vi "AsyncEngine.CANProtectionAndCounter.vi"(10 "Parameters":variant, 11 "Process":refnum<class "Process.lvclass">) -> ()   [LabVIEW 2015, in "Protection and Rolling Counter Addon Engine.lvlib"]
uses:
  Protection and Rolling Counter Addon Engine.lvlib
  <vilib>/NI/NIVS Inline Async API/_VS Inline Async API/Process/Process.lvclass
  Types/RT Async Engine Variables.ctl
  Types/RT Frame Settings.ctl
  Shared/Types/Exported Frame Type.ctl
  Types/RT Protection Configuration.ctl
  Shared/Types/Protection Type.ctl
  Shared/Types/InputChannelConfiguration.ctl
  Types/RT Counter Settings.ctl
  Shared/Types/Event Trigger Type.ctl
  Types/RT Data References.ctl
  <vilib>/NI/NIVS Inline Async API/_Data Access Engine/Data Access Engine/Types/Write.DVR.ctl
  <vilib>/NI/NIVS Inline Async API/_Data Access Engine/Access Type Classes/Write/Write.lvclass
  <vilib>/NI/NIVS Inline Async API/_Data Access Engine/Data Access Engine/Types/Read.DVR.ctl
  <vilib>/NI/NIVS Inline Async API/_Data Access Engine/Access Type Classes/Read/Read.lvclass
  <vilib>/NI/NIVS Inline Async API/_VS Inline Async API/Process/Process.lvclass/Process.ctl
  <vilib>/Platform/TimedLoop/XDataNode/timing_clust.ctl
  <vilib>/Platform/TimedLoop/XDataNode/nitl_modes.ctl
  <vilib>/Platform/TimedLoop/XDataNode/wakeup.ctl
  <vilib>/NI/NIVS Inline Async API/_Data Access Engine/Access Type Classes/Read/Read.lvclass/Read.ctl
  <vilib>/NI/NIVS Inline Async API/_Data Access Engine/Access Type Classes/Write/Write.lvclass/Write.ctl
  <vilib>/NI/NIVS Inline Async API/_VS Inline Async API/Process/Data Member Access/Read Data Access.vi
  <vilib>/NI/NIVS Inline Async API/_VS Inline Async API/Error Handling Process/SubVIs/Error.ConvertArray.vi
  <vilib>/NI/NIVS Inline Async API/_Data Access Engine/Data Access Engine/Methods/Data.Processes.Execute.vi
  <vilib>/NI/NIVS Inline Async API/_Data Access Engine/Data Access Engine/Methods/Write.Data.Buffer.vi
  SubVIs/Determine Transmission.vi
  SubVIs/Determine Periodic.vi
  <vilib>/NI/NIVS Inline Async API/_Data Access Engine/Data Access Engine/Methods/Write.Data.Commit.vi
  <vilib>/NI/NIVS Inline Async API/_Data Access Engine/Data Access Engine/Methods/Write.Data.vi
  <vilib>/NI/NIVS Inline Async API/_Data Access Engine/Data Access Engine/Methods/Read.Data.Detect.vi
  <vilib>/NI/NIVS Inline Async API/_Data Access Engine/Access Type Classes/Write/Write.Buffer.vi
  <vilib>/NI/NIVS Inline Async API/_Data Access Engine/Access Type Classes/Write/Write.Commit.vi
  <vilib>/NI/NIVS Inline Async API/_Data Access Engine/Access Type Classes/Write/Write.ProcessData.vi
  <vilib>/NI/NIVS Inline Async API/_Data Access Engine/Access Type Classes/Read/Read.ProcessData.Detect.vi
  <vilib>/xnet/xnet.llb/XNET Write.vi
  <vilib>/xnet/xnet.llb/XNET Write (Frame CAN).vi
  <vilib>/xnet/xnet.llb/XNET Convert.vi
  <vilib>/xnet/xnet.llb/XNET Convert (Signal to Frame CAN).vi
  <vilib>/xnet/xnet.llb/XNET Convert (Signal to Frame Raw).vi
  <vilib>/NI/NIVS Inline Async API/_Data Access Engine/Data Access Engine/Methods/Write.Lookup.vi
  <vilib>/NI/NIVS Inline Async API/_Data Access Engine/Data Access Engine/Methods/Read.Lookup.vi
  Shared/SubVIs/GUID Lookup.vi
  <vilib>/platform/TimedLoop/XDataNode/XDataNode.xnode
  <vilib>/NI/NIVS Inline Async API/_Data Access Engine/Data Access Engine/Data Access Engine.lvclass
  Shared/Protection and Rolling Counter Addon Shared.lvlib
  <vilib>/NI VeriStand/Custom Device Tools/Custom Device Utility Library/Custom Device Utility Library.lvlib
  <vilib>/Platform/TimedLoop/XDataNode/XDNodeRunTimeDep.lvlib
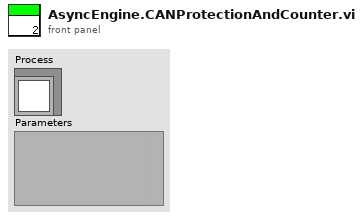
[diagram p1: front panel]
types:
  T1 = typedef "Protection and Rolling Counter Addon Engine.lvlib/RT Data References.ctl" = cluster{"ProtectionsAndCounters.Ref":T2, "Signals.Ref":T3, "Status.Ref":T2}
  T2 = typedef "Data Access Engine.lvlib/Data Access Engine.lvclass/Write.DVR.ctl" = refnum<data-value>
  T3 = typedef "Data Access Engine.lvlib/Data Access Engine.lvclass/Read.DVR.ctl" = refnum<data-value>
  T4 = typedef "Protection and Rolling Counter Addon Engine.lvlib/RT Async Engine Variables.ctl" = cluster{"Priority":i32, "CAN Session":refnum<k21>, "Frame Count":i32, "Frames":T5[], "FPGA Session":u32}
  T5 = typedef "Protection and Rolling Counter Addon Engine.lvlib/RT Frame Settings.ctl" = cluster{"Type":T6, "Frame ID":u32, "Payload Length":u32, "VS Offset":i32, "VS Length":i32, "Frame Conversion":refnum<k21>, "Frame.PrevData":dbl[], "Generation Period":u32, "Time Since Last Generation":u32, "Generation Iterations":u32, "Generation Counter":u32, "Has Protection?":bool, "Protection Configurations":T7[], "Has Counter?":bool, "Counter Configurations":T10[], "Has Disable?":bool, "Disable VS Index":i32, "Transmit Trigger":T11, "Trigger VS Index":i32}
  T6 = typedef "Protection and Rolling Counter Addon Shared.lvlib/Exported Frame Type.ctl" = enum16{"Periodic", "Event", "Periodic/Event"}
  T7 = typedef "Protection and Rolling Counter Addon Engine.lvlib/RT Protection Configuration.ctl" = cluster{"Protection Frame Index":i32, "Protection Type":T8, "Data Indeces":i32[], "Initialized Data Array":dbl[], "Check Sum Conversion":refnum<k21>, "CRC Channels":T9[], "Protection VS Index":i32}
  T8 = typedef "Protection and Rolling Counter Addon Shared.lvlib/Protection Type.ctl" = enum16{"Arb ID + Bytes Checksum with Inversion", "Arb ID + Bytes CRC with Inversion", "Reversed Raw Signal Checksum with Inversion"}
  T9 = typedef "Protection and Rolling Counter Addon Shared.lvlib/InputChannelConfiguration.ctl" = cluster{"Start Bit":i32, "Name":string, "Number of bits":i32, "Scale":dbl, "Offset":dbl, "Data Type":u32}
  T10 = typedef "Protection and Rolling Counter Addon Engine.lvlib/RT Counter Settings.ctl" = cluster{"Counter Frame Index":i32, "Max Count":dbl, "Counter VS Index":i32}
  T11 = typedef "Protection and Rolling Counter Addon Shared.lvlib/Event Trigger Type.ctl" = enum16{"Channel value change", "Trigger channel (not zero)", "Channel value change or trigger channel (not zero)", "Trigger channel (any value change)", "Channel value change or trigger channel (any value change)"}
  T12 = typedef "XDNodeRunTimeDep.lvlib/timing_clust.ctl" = cluster{"Expected End [f-1]":u64, "Actual End [f-1]":u64, "Finished Late? [f-1]":bool, "Expected End [i-1]":u64, "Actual End [i-1]":u64, "Finished Late? [i-1]":bool, "Expected Start [i]":u64, "Actual Start [i]":u64, "Expected Start [f]":u64, "Actual Start [f]":u64, "Source Name":string, "Structure Name":string, "Period":i64, "Deadline":i64, "Offset":i64, "Start":i64, "Priority":i32, "Timeout":i32, "Mode":T13, "Wakeup Reason":T14, "Error":errorcluster, "Source Type":string, "Secondary Source Type":string, "Global End Time":u64, "Global Start Time":u64, "Frame Duration":u64, "Iteration Duration":u64, "Assigned CPU":i32, "I/O Scan Engine Mode":u32}
  T13 = typedef "XDNodeRunTimeDep.lvlib/nitl_modes.ctl" = enum32{"No Change", "Process missed periods, maintain original phase", "Discard missed periods, maintain original phase", "Process missed periods, ignore original phase", "Discard missed periods, ignore original phase"}
  T14 = typedef "XDNodeRunTimeDep.lvlib/wakeup.ctl" = enum32{"Normal", "Aborted", "Asynchronous wakeup", "Timing source error", "Timed loop error", "Timeout"}
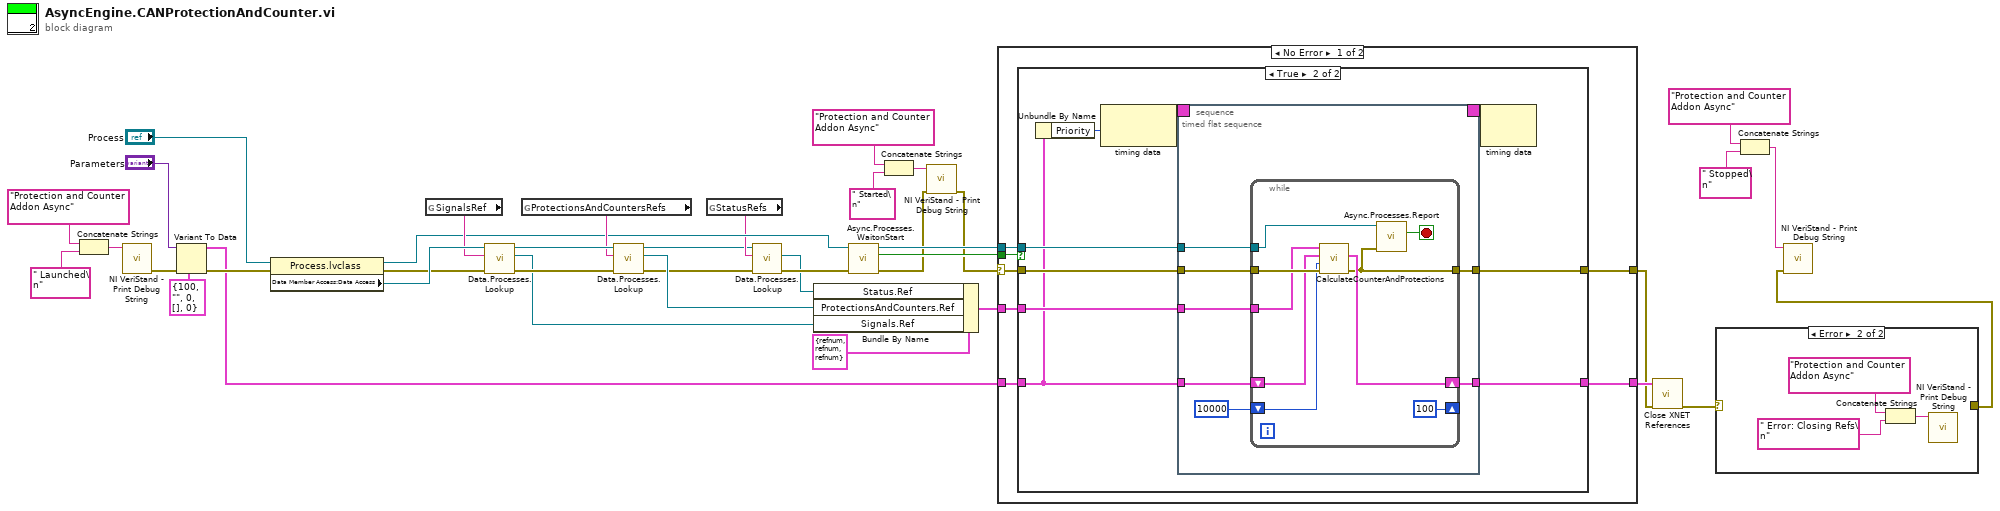
[diagram p0: block diagram]
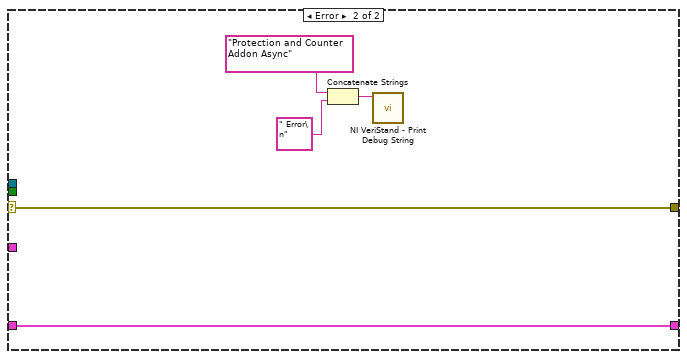
[diagram p4: hidden frame]
diagram:
  n1 = Concatenate Strings("Protection and Counter Addon Async" ("Debug String"), " Launched\n" ("string")) -> (w34:string)
  n2 = call <vilib>:"NI VeriStand - Print Debug String.vi"("Message"=w34) -> ("error out"=w32:errorcluster)  [unwired: 10 in]
  n3 = Variant To Data(error in=w32, type=T4 {"Priority"=100, "CAN Session"="", "Frame Count"=0, "Frames"=[], "FPGA Session"=0} ("RT Configuration"), Variant="Parameters") -> (data=w31:T4, error out=w37:errorcluster)
  n4 = property class="Process.lvclass"(reference="Process", error in=w37) -> (reference out=w24:refnum<class "Process.lvclass">, error out=w28:errorcluster, "Data Member Access:Data Access"=w30:refnum<class "Data Access Engine.lvclass">)
  n5 = global read "GUID Lookup.vi" "SignalsRef"() -> (w26:string)
  n6 = call-poly <vilib>:"Data.Processes.Lookup.vi"("error in (no error)"=w28, "Name"=w26, "Data Access API in"=w30) -> ("error out"=w27:errorcluster, "Ref"=w22:T3, "Data Access API out"=w29:refnum<class "Data Access Engine.lvclass">)  [unwired: 5 in, 1 out]
  n7 = global read "GUID Lookup.vi" "ProtectionsAndCountersRefs"() -> (w25:string)
  n8 = call-poly <vilib>:"Data.Processes.Lookup.vi"("error in (no error)"=w27, "Name"=w25, "Data Access API in"=w29) -> ("error out"=w15:errorcluster, "Ref"=w21:T2, "Data Access API out"=w16:refnum<class "Data Access Engine.lvclass">)  [unwired: 5 in, 1 out]
  n9 = global read "GUID Lookup.vi" "StatusRefs"() -> (w17:string)
  n10 = call-poly <vilib>:"Data.Processes.Lookup.vi"("error in (no error)"=w15, "Name"=w17, "Data Access API in"=w16) -> ("error out"=w14:errorcluster, "Ref"=w13:T2)  [unwired: 5 in, 2 out]
  n11 = Bundle By Name(cluster=T1 {"ProtectionsAndCounters.Ref"=refnum, "Signals.Ref"=refnum, "Status.Ref"=refnum}, "Status.Ref"=w13, "ProtectionsAndCounters.Ref"=w21, "Signals.Ref"=w22) -> (w18:T1)
  n12 = call <vilib>:"Async.Processes.WaitonStart.vi"("error in (no error)"=w14, "Process"=w24) -> ("error out"=w9:errorcluster, "Execute"=w19:bool, "Process out"=w23:refnum<class "Process.lvclass">)  [unwired: 7 in]
  n13 = Concatenate Strings("Protection and Counter Addon Async" ("Debug String"), " Started\n" ("string")) -> (w11:string)
  n14 = call <vilib>:"NI VeriStand - Print Debug String.vi"("error in (no error)"=w9, "Message"=w11) -> ("error out"=w8:errorcluster)  [unwired: 9 in]
  n15 = case shown="No Error" w8 {
    selector: w8 -> [w42 w90]
    tunnel: w23 -> [w46 _]
    tunnel: w19 -> [w45 _]
    tunnel: w31 -> [w44 w86]
    tunnel: w18 -> [w43 _]
    tunnel: [w41 w90] -> w2
    tunnel: [w40 w86] -> w4
    frame No Error {
      n16 = case shown="True" w45 {
        tunnel: w46 -> [_ w57]
        tunnel: w44 -> [w47 w52]
        tunnel: w43 -> [_ w56]
        tunnel: w42 -> [w48 w55]
        tunnel: [w48 w54] -> w41
        tunnel: [w47 w53] -> w40
        frame False {
        }
        frame True {
          n17 = Unbundle By Name(w52) -> ("Priority"=w49:i32)
          n18 = node-c288(w49) -> (w51:T12)
          n19 = timed-sequence {
            timing: w51 -> [_]
            timing-out: [_] -> w50
            tunnel: w57 -> [w58]
            tunnel: w52 -> [w61]
            tunnel: w56 -> [w60]
            tunnel: w55 -> [w59]
            tunnel: [w63] -> w54
            tunnel: [w62] -> w53
            n20 = timed-flat-sequence {
              tunnel: [w65] -> w63
              tunnel: [w66] -> w62
              tunnel: w61 -> [w69]
              tunnel: w60 -> [w64]
              tunnel: w59 -> [w68]
              tunnel: w58 -> [w67]
              n21 = while {
                tunnel: w67 -> [w79]
                tunnel: w64 -> [w74]
                tunnel: w68 -> [w78]
                shift-right: [w75] -> w66
                shift-left: w69 -> [w77]
                tunnel: [w73] -> w65
                shift-right: [100 ("timeout ms")] -> _
                shift-left: 10000 ("timeout ms") -> [w72]
                stop <- w76 stop-if-true
                n22 = call "CalculateCounterAndProtections.vi"("error in (no error)"=w78, "timeout ms"=w72, "Async Settings"=w77, "Data Refs"=w74) -> ("error out"=w73:errorcluster, "Async Settings"=w75:T4)  [unwired: 6 in]
                n23 = call <vilib>:"Async.Processes.Report.vi"("Error"=w73, "Process in"=w79) -> ("Stop"=w76:bool)  [unwired: 8 in, 1 out]
              }
            }
          }
          n24 = node-c288(w50) -> ()  [unwired: 1 out]
        }
      }
    }
    frame Error {
      n25 = Concatenate Strings("Protection and Counter Addon Async" ("Debug String"), " Error\n" ("string")) -> (w88:string)
      n26 = call <vilib>:"NI VeriStand - Print Debug String.vi"("Message"=w88) -> ()  [unwired: 10 in, 1 out]
    }
  }
  n27 = call "Close XNET References.vi"("error in (no error)"=w2, "RT Configuration"=w4) -> ("error out"=w3:errorcluster)  [unwired: 9 in]
  n28 = case shown="Error" w3 {
    selector: w3 -> [w91 _]
    tunnel: [w91 _] -> w1
    frame No Error {
    }
    frame Error {
      n29 = Concatenate Strings("Protection and Counter Addon Async" ("Debug String"), " Error: Closing Refs\n" ("string")) -> (w93:string)
      n30 = call <vilib>:"NI VeriStand - Print Debug String.vi"("Message"=w93) -> ()  [unwired: 10 in, 1 out]
    }
  }
  n31 = Concatenate Strings("Protection and Counter Addon Async" ("Debug String"), " Stopped\n" ("string")) -> (w6:string)
  n32 = call <vilib>:"NI VeriStand - Print Debug String.vi"("error in (no error)"=w1, "Message"=w6) -> ()  [unwired: 9 in, 1 out]
